vi "Create Resources (AXI4-Lite Address Space).vi"(0 "niInstr AXI4-Lite address space v1 FPGA in":refnum<class "niInstr AXI4-Lite Address Space v1 FPGA.lvclass">, 5 "address space size":u32, 7 "address space uid":u16) -> (4 "niInstr AXI4-Lite address space v1 FPGA out":refnum<class "niInstr AXI4-Lite Address Space v1 FPGA.lvclass">)   [LabVIEW 2015, in "niInstr AXI4-Lite Address Space v1 FPGA.lvclass"]
doc: "<B>Input Parameters</B>\n\n<B>niInstr AXI4-Lite address space v1 FPGA in</B> is the AXI4-Lite address space to use.\n\n<B>Output Parameters</B>\n\n<B>niInstr AXI4-Lite address space v1 FPGA out</B> passes a reference to the AXI4-Lite Address space to the next VI."
uses:
  <instrlib>/_niInstr/CLIP Adapters/v1/FPGA/AXI4-Lite/Address Space/niInstr AXI4-Lite Address Space v1 FPGA.lvclass
  <instrlib>/_niInstr/Instruction Framework/v1/FPGA/Typedefs/Address Map Element.ctl
  <instrlib>/_niInstr/CLIP Adapters/v1/FPGA/AXI4-Lite/Address Space/niInstr AXI4-Lite Address Space v1 FPGA.lvclass/niInstr AXI4-Lite Address Space v1 FPGA.ctl
  <instrlib>/_niInstr/Instruction Framework/v1/FPGA/Typedefs/niInstr Instruction Framework v1 FPGA.lvlib
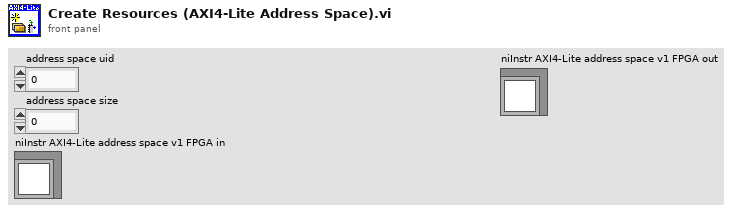
[diagram p1: front panel]
types:
  T1 = typedef "niInstr Instruction Framework v1 FPGA.lvlib/Address Map Element.ctl" = cluster{"UID":u16, "version":u16, "oldest compatible version":u16, "instance":u8, "number of children":u8, "offset":u32}
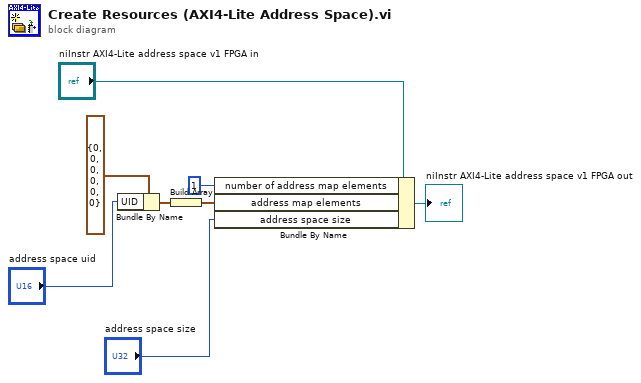
[diagram p0: block diagram]
diagram:
  n1 = Bundle By Name(cluster=T1 {"UID"=0, "version"=0, "oldest compatible version"=0, "instance"=0, "number of children"=0, "offset"=0} ("address map element"), "UID"="address space uid") -> (w5:T1)
  n2 = Build Array(w5) -> (w2:T1[])
  n3 = Bundle By Name(cluster="niInstr AXI4-Lite address space v1 FPGA in", "number of address map elements"=u32 1, "address map elements"=w2, "address space size"="address space size") -> (→"niInstr AXI4-Lite address space v1 FPGA out":refnum<class "niInstr AXI4-Lite Address Space v1 FPGA.lvclass">)
